vi "GetNet-Client Check Network Parameters.vi"(8 "error in (no error)":errorcluster, 9 "Timeout":i32, 10 "Port":u16, 11 "IP":string) -> (0 "error out":errorcluster)   [LabVIEW 2020, in "GenNet-Client.lvlib"]
doc: "Checks the connection parameters for valid settings (IP address, port number)\n\n____\nHAMPEL SOFTWARE ENGINEERING v3.8.0 (2023-12-18 14:41)"
uses:
  GenNet-Client.lvlib
  hse-networking/hse-network.lvlib
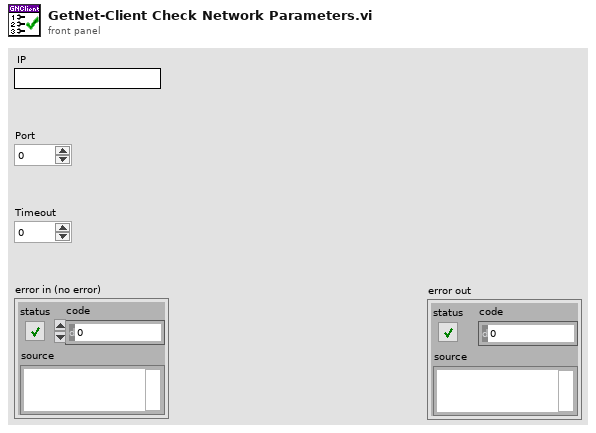
[diagram p1: front panel]
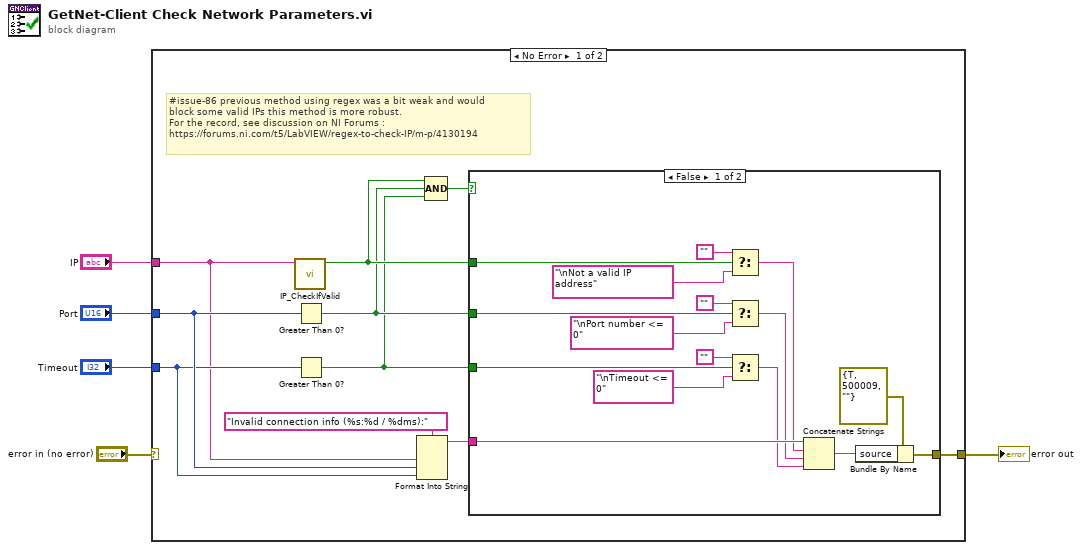
[diagram p0: block diagram]
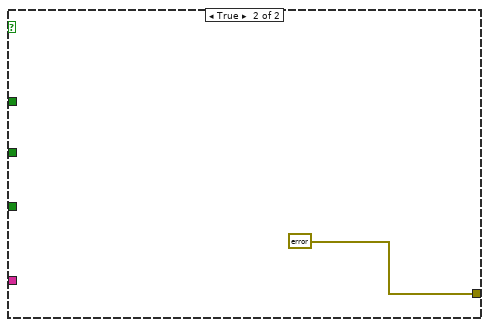
[diagram p2: hidden frame]
diagram:
  n1 = case shown="No Error" "error in (no error)" {
    selector: "error in (no error)" -> [_ w33]
    tunnel: [w14 w33] -> w4
    tunnel: "IP" -> [w9 _]
    tunnel: "Port" -> [w11 _]
    tunnel: "Timeout" -> [w10 _]
    frame No Error {
      # "#issue-86 previous method using regex was a bit weak and would \nblock some valid IPs this method is more robust.\nFor the record, see discussion on NI Forums : \nhttps://forums.ni.com/t5/LabVIEW/regex-to-check-IP/m-p/4130194"
      n2 = call "IP_CheckIfValid.vi"("IP"=w9) -> ("Valid IP"=w8:bool)  [unwired: 10 in]
      n3 = Greater Than 0?(x=w11) -> (x > 0?=w7:bool)
      n4 = Greater Than 0?(x=w10) -> (x > 0?=w6:bool)
      n5 = Format Into String(format string="Invalid connection info (%s:%d / %dms):", w9, w11, w10) -> (resulting string=w12:string)  [unwired: 2 in, 1 out]
      n6 = Compound Arithmetic op=AND(w8, w7, w6) -> (w15:bool)
      n7 = case shown="False" w15 {
        tunnel: [w29 errorcluster {"status"=FALSE, "code"=0, "source"=""} ("error IO")] -> w14
        tunnel: w12 -> [w30 _]
        tunnel: w8 -> [w28 _]
        tunnel: w7 -> [w20 _]
        tunnel: w6 -> [w19 _]
        frame False {
          n8 = Select(t="", s=w28, f="\nNot a valid IP address" ("format string")) -> (s? t:f=w23:string)
          n9 = Select(t="", s=w20, f="\nPort number <= 0" ("format string")) -> (s? t:f=w22:string)
          n10 = Select(t="", s=w19, f="\nTimeout <= 0" ("format string")) -> (s? t:f=w21:string)
          n11 = Concatenate Strings(w30, w23, w22, w21) -> (w24:string)
          n12 = Bundle By Name(cluster=errorcluster {"status"=TRUE, "code"=500009, "source"=""} ("error IO"), "source"=w24) -> (w29:errorcluster)
        }
        frame True {
        }
      }
    }
    frame Error {
    }
  }
  "error out" <- w4
